vi "TSM SSC Digital PPMU Measure Voltage.vi"(0 "Digital TSM In":T1, 11 "error in":errorcluster) -> (4 "Digital TSM Out":T1, 6 "Per-Site Per-Pin Measurements (V)":dbl[][](array[numeric]), 15 "error out":errorcluster)   [LabVIEW 2020]
doc: "Instructs the PPMU to measure voltage on the specified pin(s) and pin group(s) and returns per-site per-pin voltage measurements."
uses:
  TSM/TSM SSC Digital.ctl
  <vilib>/NI_TestStand_SemiconductorModule/NI_TestStand_Semiconductor_Module.lvlibp/PinMap/Digital Pattern/PinQueryContext/DigitalPatternPinQueryContext.lvclass
  SSC Digital/SSC Digital.ctl
  <instrlib>/niDigital/niDigital.llb/niDigital Measurement Type.ctl
  33e6599e-1cf0-4320-8f9c-b6d8077a7b37.vi
  Shared SubVIs/Channel List to Pins.vi
  Shared SubVIs/Trim Whitespace [Inlined].vi
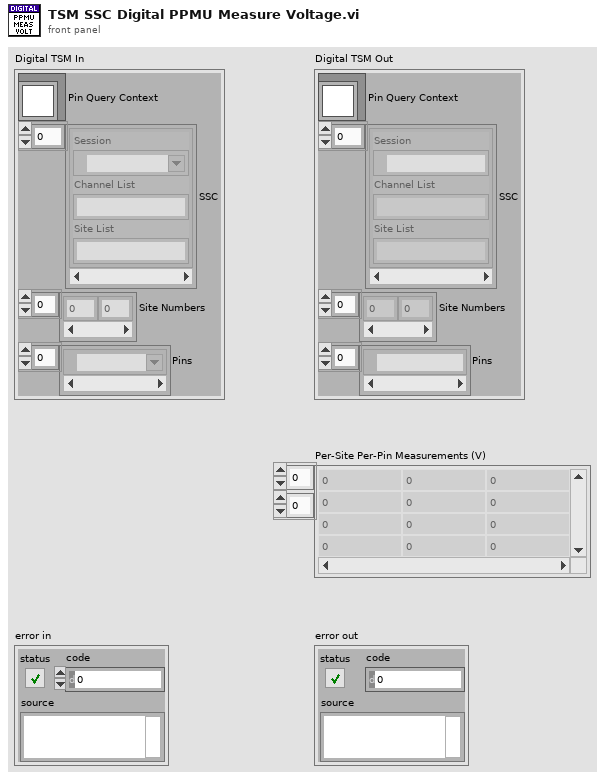
[diagram p1: front panel]
types:
  T1 = typedef "TSM SSC Digital.ctl" = cluster{"Pin Query Context":refnum<class "DigitalPatternPinQueryContext.lvclass">, "SSC":T2[], "Site Numbers":i32[], "Pins":tag[]}
  T2 = typedef "SSC Digital.ctl" = cluster{"Session":refnum<k15>, "Channel List":string, "Site List":string}
  T3 = typedef "niDigital Measurement Type.ctl" = i32
  T4 = typedef "Digital 2D Location Array in a Cluster.ctl" = cluster{"Digital 2D Location Array":T5[]}
  T5 = typedef "Digital 2D Location.ctl" = cluster{"Row":i32, "Col":i32}
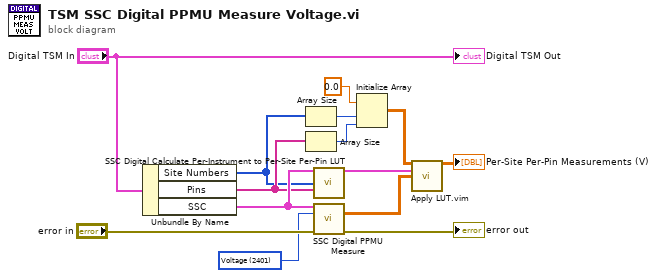
[diagram p0: block diagram]
diagram:
  w1 = T3 2401 items=["Voltage"=2401, "Current"=2400] ("measurement type")
  n1 = Unbundle By Name("Digital TSM In") -> ("Site Numbers"=w5:i32[], "Pins"=w6:tag[], "SSC"=w13:T2[])
  n2 = Array Size(array=w5) -> (size(s)=w2:i32)
  n3 = Array Size(array=w6) -> (size(s)=w3:i32)
  n4 = call "SSC Digital Calculate Per-Instrument to Per-Site Per-Pin LUT.vi"("Digital SSC In"=w13, "Sites"=w5, "Pins"=w6) -> ("Per-Instrument to Per-Site Per-Pin LUT"=w4:T4[])  [unwired: 12 in]
  n5 = call "SSC Digital PPMU Measure.vi"("Digital SSC in"=w13, "Measurement Type"=w1, "error in"="error in") -> ("Per-Instrument Measurements"=w12:dbl[][], "error out"=→"error out":errorcluster)  [unwired: 10 in, 1 out]
  n6 = Initialize Array(0.0 ("element"), w2, w3) -> (w7:dbl[][])
  n7 = call "Apply LUT.vim"("Initialized Array"=w7, "LUT"=w4, "Results to Apply LUT to"=w12) -> ("Array Out"=→"Per-Site Per-Pin Measurements (V)":dbl[][])  [unwired: 12 in]
  "Digital TSM Out" <- "Digital TSM In"
